vi "操作信息显示.vi"() -> ()   [LabVIEW 2013]
panel:
  out "String":string
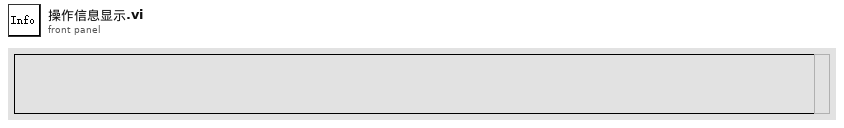
[diagram p1: front panel]
types:
  T1 = enum16{"open", "replace", "create", "open or create", "replace or create", "replace or create with confirmation"}
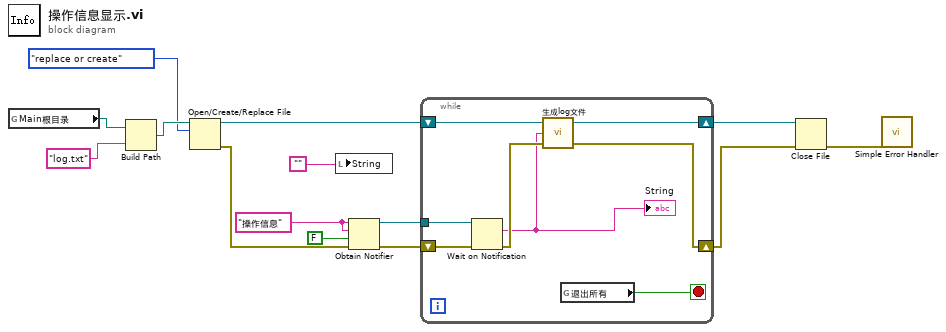
[diagram p0: block diagram]
diagram:
  w14 = "操作信息"
  n1 = global read "Main根目录.vi" "Main根目录"() -> (w9:path)
  n2 = Build Path(base path=w9, name or relative path="log.txt") -> (appended path=w8:path)
  n3 = Open/Create/Replace File(file path (use dialog)=w8, operation (0:open)=T1."replace or create") -> (refnum out=w6:refnum<file>, error out=w1:errorcluster)  [unwired: 4 in, 1 out]
  n4 = local write "String"("") -> ()
  n5 = Obtain Notifier(name (unnamed)=w14, notification data type=w14, create if not found? (T)=FALSE, error in (no error)=w1) -> (notifier out=w12:refnum<notifier>, error out=w4:errorcluster)  [unwired: 1 out]
  n6 = while {
    tunnel: w12 -> [w22]
    shift-right: [w18] -> w5
    shift-left: w6 -> [w19]
    shift-right: [w16] -> w3
    shift-left: w4 -> [w17]
    stop <- w15 stop-if-true
    n7 = Wait on Notification(notifier=w22, error in (no error)=w17) -> (notification=w20:string, error out=w21:errorcluster)  [unwired: 2 in, 2 out]
    "String" <- w20
    n8 = call "生成log文件.vi"("error in (no error)"=w21, "信息"=w20, "refnum in"=w19) -> ("error out"=w16:errorcluster, "refnum out"=w18:refnum<file>)  [unwired: 1 out]
    n9 = global read "退出所有.vi" "退出所有"() -> (w15:bool)
  }
  n10 = Close File(refnum=w5, error in=w3) -> (error out=w2:errorcluster)  [unwired: 1 out]
  n11 = call <vilib>:"Simple Error Handler.vi"("error in (no error)"=w2) -> ()  [unwired: 4 in, 5 out]
